vi "Pre Launch Init.vi"(11 "Unit_Test_NI6008 in":refnum<class "Unit_Test_NI6008.lvclass">) -> (0 "error out":errorcluster, 3 "Unit_Test_NI6008 out":refnum<class "Unit_Test_NI6008.lvclass">)   [LabVIEW 2020, in "Unit_Test_NI6008.lvlib" / "Unit_Test_NI6008.lvclass"]
doc: "(<B>Filename</B>: Actor Framework.lvlib:Actor.lvclass:Pre Launch Init.vi)\n\nDefines behavior that occurs after the Launch Nested Actor method is invoked but before the actor's Actor Core method begins running.\n\nBy default, this method does nothing. A descendant class may override it to define behavior."
uses:
  Unit_Test_NI6008.lvclass
  <vilib>/ActorFramework/Actor/Actor.lvclass
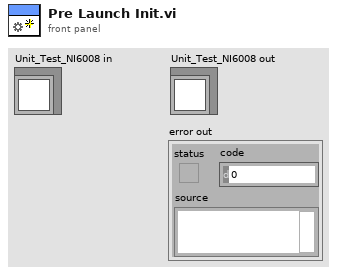
[diagram p1: front panel]
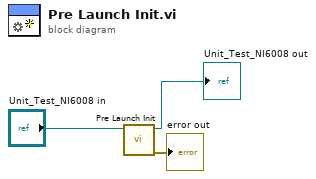
[diagram p0: block diagram]
diagram:
  n1 = call-parent "Pre Launch Init.vi"("Actor in"="Unit_Test_NI6008 in") -> ("error out"=→"error out":errorcluster, "Actor out"=→"Unit_Test_NI6008 out":refnum<class "Unit_Test_NI6008.lvclass">)  [unwired: 9 in]
